vi "Write Test Result.vi"(8 "error in (no error)":errorcluster, 10 "Test Result":refnum<class "Test Result.lvclass">, 11 "Test Report in":refnum<class "Test Report.lvclass">) -> (0 "error out":errorcluster, 3 "Test Report out":refnum<class "Test Report.lvclass">)   [LabVIEW 2009, in "Caraya.lvlib" / "Test Report.lvclass"]
uses:
  Test Report.lvclass
  Test Result/Test Result.lvclass
  Test Report.lvclass/Test Report.ctl
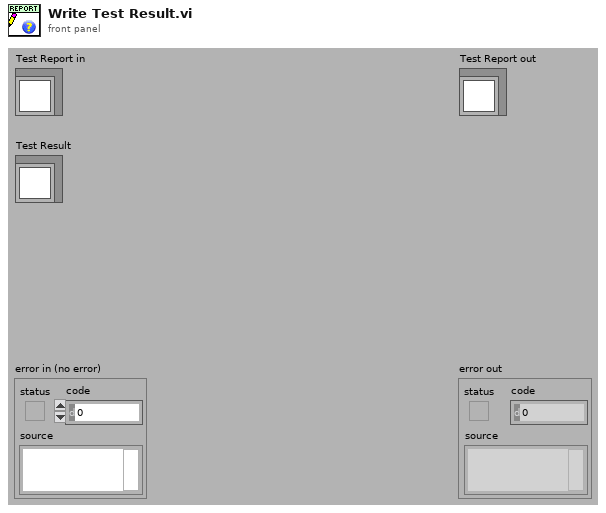
[diagram p1: front panel]
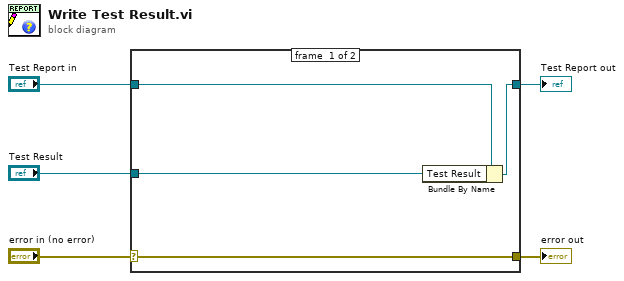
[diagram p0: block diagram]
diagram:
  n1 = case shown="No Error" "error in (no error)" {
    selector: "error in (no error)" -> [w9 w10]
    tunnel: [w9 w10] -> w4
    tunnel: [w7 w11] -> w2
    tunnel: "Test Report in" -> [w8 w11]
    tunnel: "Test Result" -> [w6 _]
    frame #0 {
      n2 = Bundle By Name(cluster=w8, "Test Result"=w6) -> (w7:refnum<class "Test Report.lvclass">)
    }
    frame #1 {
    }
  }
  "error out" <- w4
  "Test Report out" <- w2
